vi "Element in queue.vi"(11 "queue":T1) -> (2 "Ready to read":bool, 3 "queue out":T1)   [LabVIEW 2016]
uses:
  Program Files (x86)/National Instruments/LabVIEW 2016/examples/robotics/EPOS2 CANOpen Driver/Low Level VIs/Typedefs/Write Queue.ctl
  Program Files (x86)/National Instruments/LabVIEW 2016/examples/robotics/EPOS2 CANOpen Driver/Low Level VIs/Typedefs/FPGA CAN Frame Cluster.ctl
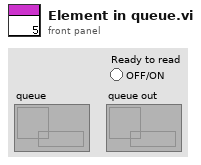
[diagram p1: front panel]
types:
  T1 = typedef "Write Queue.ctl" = refnum<queue>
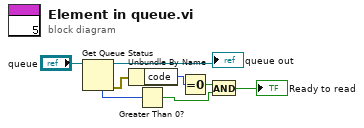
[diagram p0: block diagram]
diagram:
  n1 = Get Queue Status(queue="queue") -> (queue out=→"queue out":T1, error out=w8:errorcluster, # elements in queue=w6:i32)  [unwired: 2 in, 5 out]
  n2 = Unbundle By Name(w8) -> ("code"=w7:i32)
  n3 = Greater Than 0?(x=w6) -> (x > 0?=w4:bool)
  n4 = Equal To 0?(x=w7) -> (x = 0?=w5:bool)
  n5 = And(x=w5, y=w4) -> (x .and. y?=→"Ready to read":bool)
